vi "ClimberOutput.vi"   [LabVIEW 2019]
uses:
  refnums.vi
  outputs.vi
  6fe8d475-cc12-459e-ab35-a48b35134930.vi
  dsdata.vi
  <vilib>/Rock Robotics/WPI/Solenoid/WPI_SolenoidValue.ctl
  <vilib>/Rock Robotics/WPI/Solenoid/WPI_SolenoidSetEnum.vi
  c95c97c9-e502-477e-b9e3-4143b710e072.vi
  GRNF_GenericSolenoid.vi
types:
  T1 = typedef "WPI_SolenoidDevRef.ctl" = cluster{"DevStatus":errorcluster, "Pneumatics Control Module":u8, "Forward Solenoid Channel":T2, "Reverse Solenoid Channel":T2}
  T2 = typedef "WPI_SolenoidChannel.ctl" = enum8{"Solenoid 0", "Solenoid 1", "Solenoid 2", "Solenoid 3", "Solenoid 4", "Solenoid 5", "Solenoid 6", "Solenoid 7", "Invalid"}
  T3 = typedef "WPI_DriverStationRobotMode2.ctl" = enum16{"Autonomous Disabled", "Autonomous Enabled", "Teleop Disabled", "Teleop Enabled", "Disconnected", "Finish", "Test Disabled", "Test Enabled", "Emergency Stopped"}
  T4 = typedef "WPI_SolenoidValue.ctl" = enum16{"Off", "On", "Forward", "Reverse"}
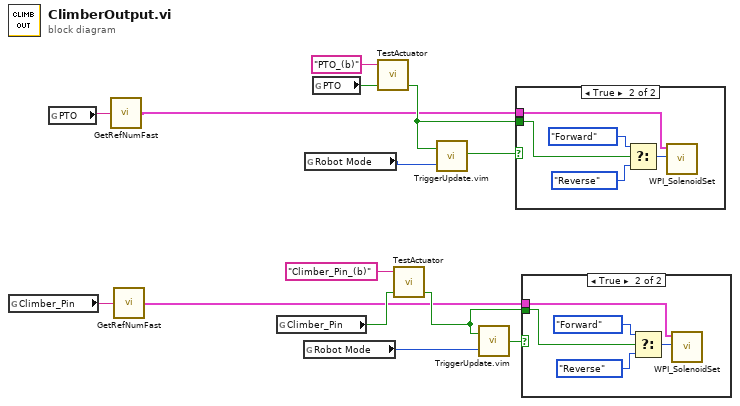
[diagram p0: block diagram]
diagram:
  n1 = global read "refnums.vi" "Climber_Pin"() -> (w1:string)
  n2 = global read "refnums.vi" "PTO"() -> (w2:string)
  n3 = call-poly "GetRefNumFast.vi"("RefNum Name"=w2) -> ("Device Reference"=w4:T1)
  n4 = call-poly "GetRefNumFast.vi"("RefNum Name"=w1) -> ("Device Reference"=w3:T1)
  n5 = global read "outputs.vi" "Climber_Pin"() -> (w13:bool)
  n6 = global read "dsdata.vi" "Robot Mode"() -> (w7:T3)
  n7 = global read "dsdata.vi" "Robot Mode"() -> (w5:T3)
  n8 = global read "outputs.vi" "PTO"() -> (w10:bool)
  n9 = call "TestActuator.vi"("Input_Value_Boolean"=w10, "Actuator_Name"="PTO_(b)") -> ("Output_Value_Boolean"=w11:bool)  [unwired: 1 in, 2 out]
  n10 = call "TestActuator.vi"("Input_Value_Boolean"=w13, "Actuator_Name"="Climber_Pin_(b)") -> ("Output_Value_Boolean"=w14:bool)  [unwired: 1 in, 2 out]
  n11 = call "TriggerUpdate.vim"("Robot Mode"=w5, "Trigger"=w11) -> ("Update"=w6:bool)
  n12 = call "TriggerUpdate.vim"("Robot Mode"=w7, "Trigger"=w14) -> ("Update"=w8:bool)
  n13 = case shown="True" w6 {
    tunnel: w11 -> [_ w16]
    tunnel: w4 -> [_ w15]
    frame False {
    }
    frame True {
      n14 = Select(t=WPI_SolenoidValue."Forward" ("Value"), s=w16, f=WPI_SolenoidValue."Reverse" ("Value")) -> (s? t:f=w19:T4)
      n15 = call-poly <vilib>:"WPI_SolenoidSet.vi"("Value"=w19, "SolenoidDevRef"=w15) -> ()  [unwired: 8 in, 2 out]
    }
  }
  n16 = case shown="True" w8 {
    tunnel: w14 -> [_ w21]
    tunnel: w3 -> [_ w20]
    frame False {
    }
    frame True {
      n17 = Select(t=WPI_SolenoidValue."Forward" ("Value"), s=w21, f=WPI_SolenoidValue."Reverse" ("Value")) -> (s? t:f=w24:T4)
      n18 = call-poly <vilib>:"WPI_SolenoidSet.vi"("Value"=w24, "SolenoidDevRef"=w20) -> ()  [unwired: 8 in, 2 out]
    }
  }
